vi "Esercitazione 7 - Signal Generation.vi"() -> ()   [LabVIEW 2018]
uses:
  <vilib>/Analysis/4window.llb/windowTd.ctl
  <vilib>/measure/maspectr.llb/FFT Spectrum (Mag-Phase) for 1 Chan.vi
  <vilib>/measure/NI_MABase.lvlib
  <vilib>/measure/NI_MAPro.lvlib
  <vilib>/Analysis/NI_AALPro.lvlib
panel:
  out "df":dbl
  out "f0":dbl
  in  "window":T1=1 items=["Rectangle"=0, "Hanning"=1, "Hamming"=2, "Blackman-Harris"=3, "Exact Blackman"=4, "Blackman"=5, "Flat Top"=6, "4 Term B-Harris "=7, "7 Term B-Harris"=8, "Low Sidelobe"=9, "Blackman Nuttall"=11, "Triangle"=30, "Bartlett-Hanning"=31, "Bohman"=32, "Parzen"=33, "Welch"=34, "Kaiser"=60, "Dolph-Chebyshev"=61, "Gaussian"=62]
  out "Waveform Graph 2":dbl[](graph)
  in  "sampling info":cluster{"Fs":dbl, "#s":dbl}={"Fs"=1000.0, "#s"=1000.0} {"Fs" format="%.2p"}
  out "P val":dbl
  out "A val":dbl
  out "F val":dbl
  in  "signal type":T2(ring)
  in  "Phase":i16(knob) scale=0.0..100.0
  in  "Amplitude":i16(knob) scale=0.0..10.0
  in  "Frequency":i16(knob) scale=0.0..10.0
  out "Waveform Graph":waveform(dbl)(graph)
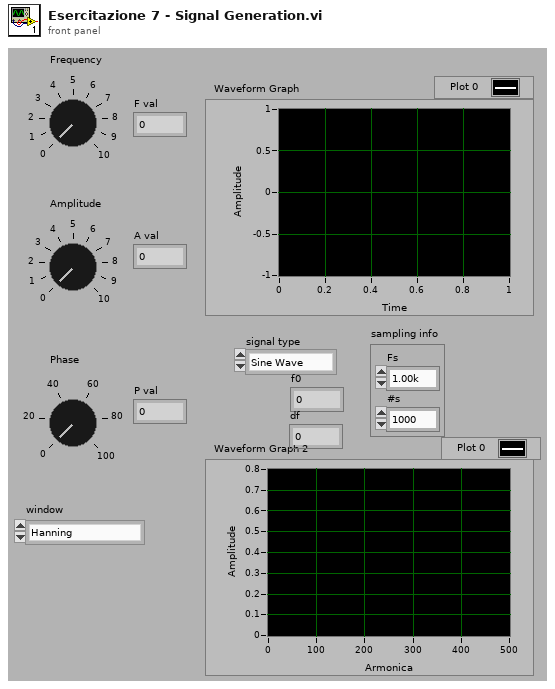
[diagram p1: front panel]
types:
  T1 = typedef "NI_AALPro.lvlib/windowTd.ctl" = u32
  T2 = enum16{"Sine Wave", "Triangle Wave", "Square Wave", "Sawtooth Wave"}
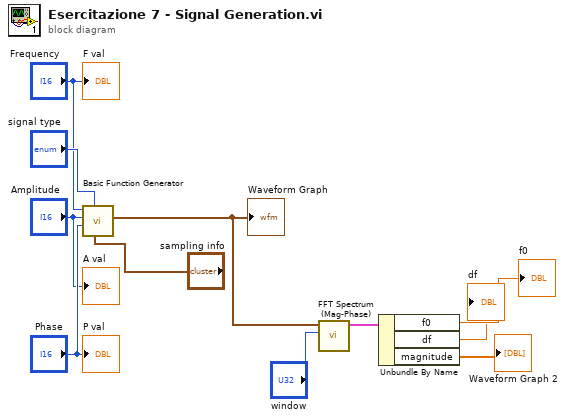
[diagram p0: block diagram]
diagram:
  n1 = call <vilib>:"Basic Function Generator.vi"("sampling info"="sampling info", "signal type"="signal type", "phase"="Phase", "amplitude"="Amplitude", "frequency"="Frequency") -> ("signal out"=w6:waveform(dbl))  [unwired: 4 in, 2 out]
  "Waveform Graph" <- w6
  n2 = call-poly <vilib>:"FFT Spectrum (Mag-Phase).vi"("window"="window", "time signal"=w6) -> ("magnitude"=w5:cluster{"f0":dbl, "df":dbl, "magnitude":dbl[]})  [unwired: 5 in, 4 out]
  n3 = Unbundle By Name(w5) -> ("f0"=→"f0":dbl, "df"=→"df":dbl, "magnitude"=→"Waveform Graph 2":dbl[])
  "F val" <- "Frequency"
  "A val" <- "Amplitude"
  "P val" <- "Phase"
